vi "PIXY rev bits.vi"(10 "SPIDevRef in":T1, 11 "SPI to Send":u8[](array[numeric])) -> (0 "error out":errorcluster, 2 "Received Data":u8[](array[numeric]), 3 "SPIDevRef out":T1)   [LabVIEW 2016]
uses:
  <vilib>/Rock Robotics/WPI/SPI/WPI_SPIDevRef.ctl
  <vilib>/Rock Robotics/SystemInterfaces/spilib/spi_bus.ctl
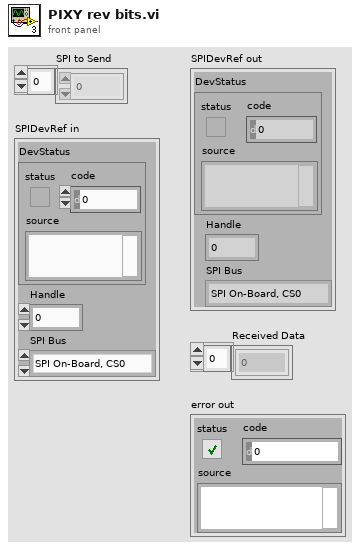
[diagram p1: front panel]
types:
  T1 = typedef "WPI_SPIDevRef.ctl" = cluster{"DevStatus":errorcluster, "Handle":i32, "SPI Bus":T2}
  T2 = typedef "spi_bus.ctl" = enum16{"SPI On-Board, CS0", "SPI On-Board, CS1", "SPI On-Board, CS2", "SPI On-Board, CS3", "SPI MXP", "Invalid"}
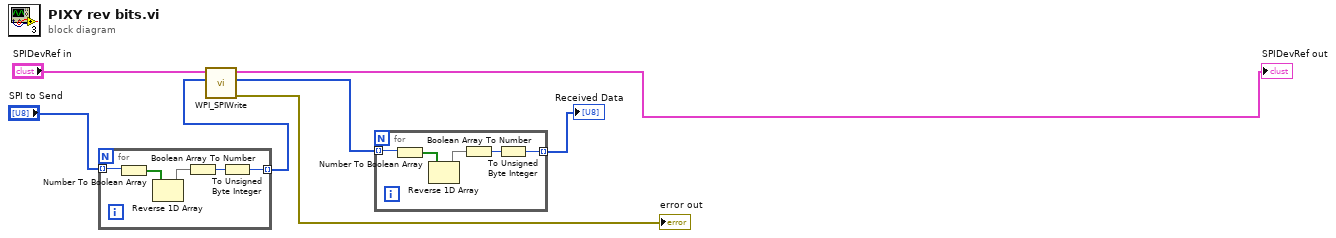
[diagram p0: block diagram]
diagram:
  n1 = for {
    tunnel: "SPI to Send" -> [w12] mode=indexing
    tunnel: [w8] -> w3 mode=indexing
    n2 = Number To Boolean Array(number=w12) -> (Boolean array=w11:bool[])
    n3 = Reverse 1D Array(array=w11) -> (reversed array=w10:bool[])
    n4 = Boolean Array To Number(Boolean array=w10) -> (number=w9:u32)
    n5 = To Unsigned Byte Integer(number=w9) -> (unsigned 8bit integer=w8:u8)
  }
  n6 = call <vilib>:"WPI_SPIWrite.vi"("Data To Send"=w3, "SPIDevRef"="SPIDevRef in") -> ("error out"=→"error out":errorcluster, "Received Data"=w1:u8[], "SPIDevRef"=→"SPIDevRef out":T1)  [unwired: 7 in]
  n7 = for {
    tunnel: w1 -> [w17] mode=indexing
    tunnel: [w13] -> w2 mode=indexing
    n8 = Number To Boolean Array(number=w17) -> (Boolean array=w16:bool[])
    n9 = Reverse 1D Array(array=w16) -> (reversed array=w15:bool[])
    n10 = Boolean Array To Number(Boolean array=w15) -> (number=w14:u32)
    n11 = To Unsigned Byte Integer(number=w14) -> (unsigned 8bit integer=w13:u8)
  }
  "Received Data" <- w2
